vi "Estimación de velocidad escribir.vi"() -> ()   [LabVIEW 2024]
uses:
  <vilib>/Instr/_visa.llb/VISA Configure Serial Port (Instr).vi
panel:
  out "VELOCIDAD":u8(knob) scale=0.0..100.0
  in  "Dato de envio":string
  out "revoluciones por minuto":dbl
  out "pulsos por segundo":dbl
  out "RPS":u8(knob) scale=0.0..20.0
  out "RPM":dbl(knob) scale=0.0..1000.0
  out "dato de pwm":string
  in  "Control de velocidad \n(+/-)":dbl(knob) scale=0.0..255.0
  out "Lectura del canal serial":string
  in  "Stop":bool
  in  "Puerto para el Arduino":refnum<visa-resource-name>
  # "VELOCIDAD DE MOTOR DC                             JUAN DAVID SOTELO\n                                                                       JERSON OSWALDO SIERRA"
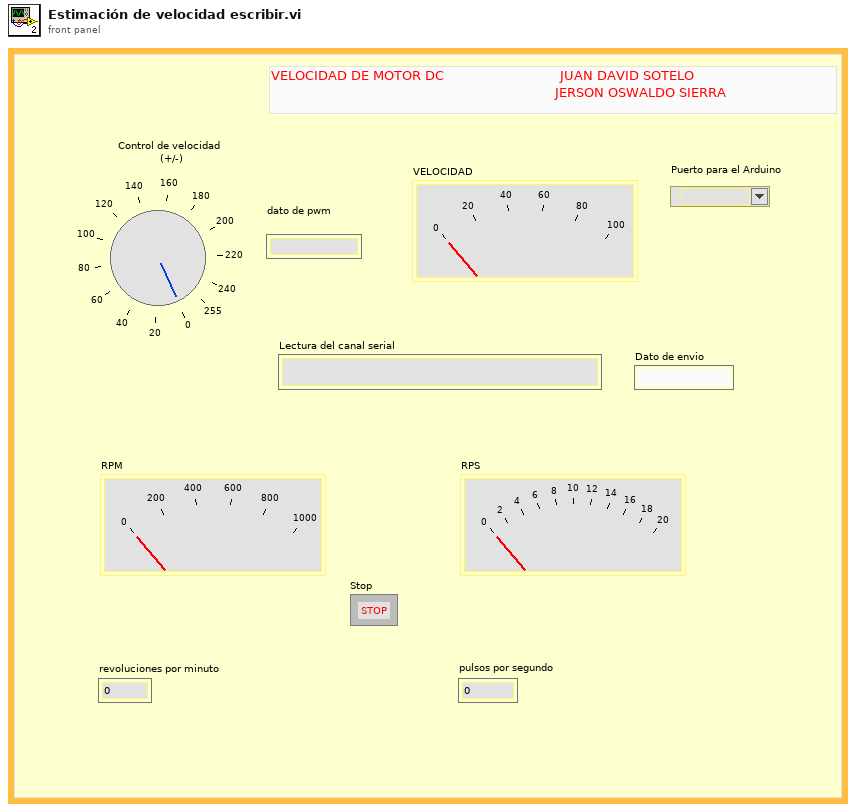
[diagram p1: front panel]
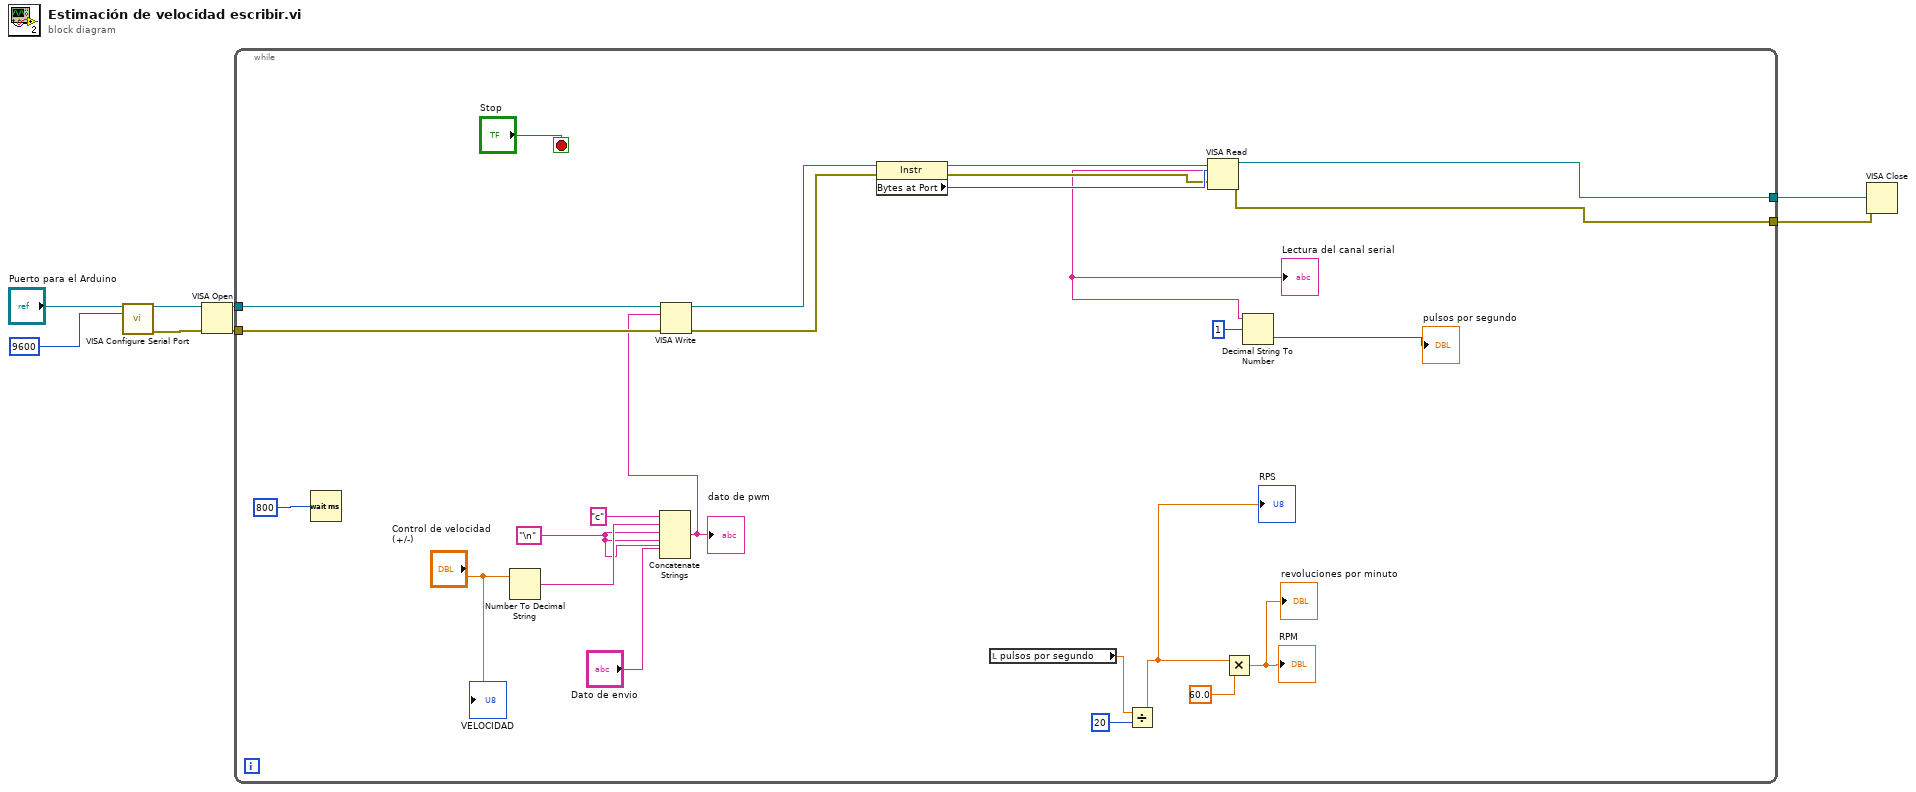
[diagram p0: block diagram]
diagram:
  n1 = call-poly "VISA Configure Serial Port"("VISA resource name"="Puerto para el Arduino", "baud rate (9600)"=u32 9600) -> ("VISA resource name out"=w6:refnum<visa-resource-name>, "error out"=w5:errorcluster)  [unwired: 12 in]
  n2 = VISA Open(error in (no error)=w5, VISA resource name=w6) -> (VISA resource name=w2:refnum<visa-resource-name>, error out=w1:errorcluster)  [unwired: 3 in]
  n3 = while {
    tunnel: [w16] -> w4
    tunnel: [w29] -> w3
    tunnel: w2 -> [w28]
    tunnel: w1 -> [w27]
    stop <- "Stop" stop-if-true
    w22 = "\n" ("write buffer")
    n4 = Wait (ms)(milliseconds to wait=u32 800) -> ()  [unwired: 1 out]
    n5 = Number To Decimal String(number="Control de velocidad \n(+/-)") -> (decimal integer string=w24:string)  [unwired: 1 in]
    n6 = Concatenate Strings("c" ("string"), w24, w22, w22, "Dato de envio", w22) -> (w13:string)
    "dato de pwm" <- w13
    n7 = VISA Write(VISA resource name=w28, write buffer=w13, error in (no error)=w27) -> (VISA resource name out=w26:refnum<visa-resource-name>, error out=w25:errorcluster)  [unwired: 1 out]
    n8 = property class="Instr"(reference=w26, error in=w25) -> (reference out=w17:refnum<visa-resource-name>, error out=w30:errorcluster, "Bytes at Port"=w31:u32)
    n9 = local read "pulsos por segundo"() -> (w11:dbl)
    n10 = Divide(x=w11, y=20) -> (x/y=w10:dbl)
    "RPS" <- w10
    n11 = VISA Read(VISA resource name=w17, byte count=w31, error in (no error)=w30) -> (VISA resource name out=w16:refnum<visa-resource-name>, read buffer=w15:string, error out=w29:errorcluster)  [unwired: 1 out]
    "Lectura del canal serial" <- w15
    n12 = Multiply(x=w10, y=60.0) -> (x*y=→"RPM" →"revoluciones por minuto":dbl)
    n13 = Decimal String To Number(string=w15, offset=1) -> (number=→"pulsos por segundo":i32)  [unwired: 1 in, 1 out]
    "VELOCIDAD" <- "Control de velocidad \n(+/-)"
  }
  n14 = VISA Close(VISA resource name=w4, error in (no error)=w3) -> ()  [unwired: 1 out]
